vi "Test-SharedVariable-WriteQueue.vi"   [LabVIEW 2014]
types:
  T1 = cluster{"试验ID":u32, "报警级别":string, "报警系统":string, "报警详情":string, "备注":string}
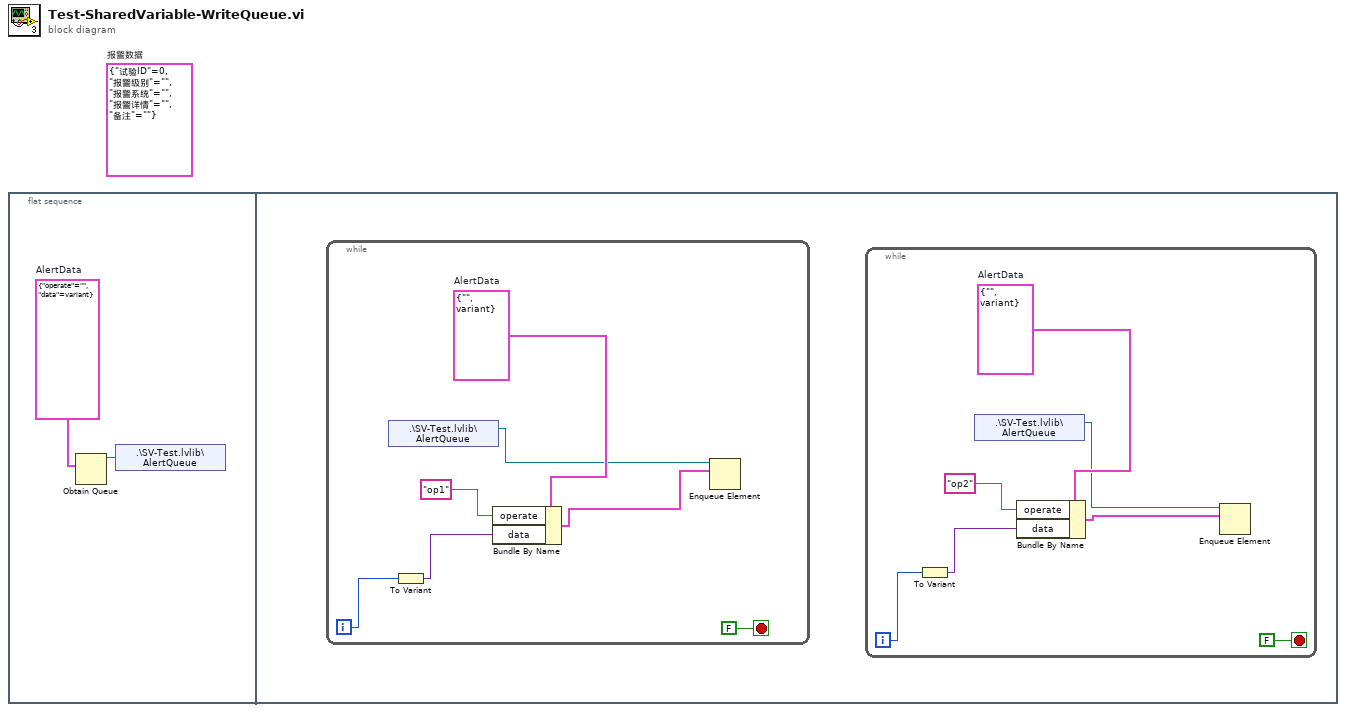
[diagram p0: block diagram]
diagram:
  (unwired) T1 {"试验ID"=0, "报警级别"="", "报警系统"="", "报警详情"="", "备注"=""}  # 报警数据
  n1 = flat-sequence {
    frame #0 {
      w2 = cluster{"operate":string, "data":variant} {"operate"="", "data"=variant}  # AlertData
      n2 = Obtain Queue(element data type=w2) -> (queue out=w1:refnum<queue>)  [unwired: 4 in, 2 out]
      n3 = shared-variable ".\\SV-Test.lvlib\\AlertQueue"(w1) -> ()  [unwired: 1 in, 1 out]
    }
    frame #1 {
      n4 = while {
        i -> [w13]
        stop <- FALSE stop-if-true
        w15 = cluster{"operate":string, "data":variant} {"operate"="", "data"=variant}  # AlertData
        n5 = shared-variable ".\\SV-Test.lvlib\\AlertQueue"() -> (w11:refnum<queue>)  [unwired: 1 in, 1 out]
        n6 = To Variant(anything=w13) -> (Variant=w12:variant)
        n7 = Bundle By Name(cluster=w15, "operate"="op1", "data"=w12) -> (w10:cluster{"operate":string, "data":variant})
        n8 = Enqueue Element(queue=w11, element=w10) -> ()  [unwired: 2 in, 3 out]
      }
      n9 = while {
        i -> [w6]
        stop <- FALSE stop-if-true
        w7 = cluster{"operate":string, "data":variant} {"operate"="", "data"=variant}  # AlertData
        n10 = To Variant(anything=w6) -> (Variant=w9:variant)
        n11 = shared-variable ".\\SV-Test.lvlib\\AlertQueue"() -> (w4:refnum<queue>)  [unwired: 1 in, 1 out]
        n12 = Bundle By Name(cluster=w7, "operate"="op2", "data"=w9) -> (w3:cluster{"operate":string, "data":variant})
        n13 = Enqueue Element(queue=w4, element=w3) -> ()  [unwired: 2 in, 3 out]
      }
    }
  }
